vi "form_send_command.vi"(11 "JSON":string) -> ()   [LabVIEW 2021]
doc: "Form for sinding a command."
uses:
  core/host_global_vars.vi
panel:
  in  "command":string
  in  "send button":bool
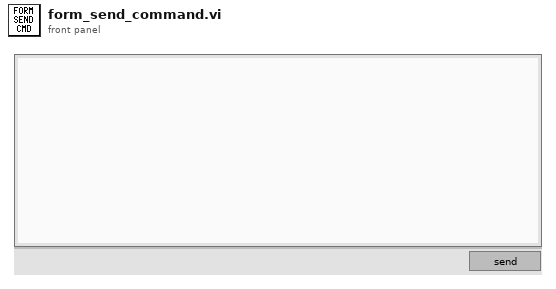
[diagram p1: front panel]
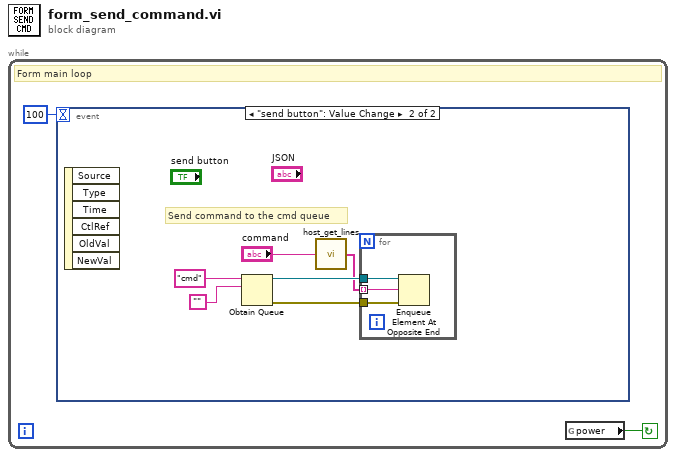
[diagram p0: block diagram]
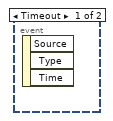
[diagram p2: hidden frame]
diagram:
  n1 = while {
    stop <- w2 continue-if-true
    # "Form main loop"
    n2 = event shown="[1] \"send button\": Value Change" {
      selector: _ -> [_ _]
      dyn-events: _ -> [_ _]
      timeout: 100 -> [_ _]
      event Timeout {
        n3 = event-data() -> ()  [unwired: 1 in, 3 out]
      }
      event "send button": Value Change {
        # "Send command to the cmd queue"
        n4 = event-data() -> ()  [unwired: 1 in, 6 out]
        n5 = Obtain Queue(name (unnamed)="cmd", element data type="") -> (queue out=w6:refnum<queue>, error out=w5:errorcluster)  [unwired: 3 in, 1 out]
        n6 = call "host_get_lines.vi"("in"="command") -> ("out"=w3:string[])
        n7 = for {
          tunnel: w6 -> [w11]
          tunnel: w5 -> [w10]
          tunnel: w3 -> [w9] mode=indexing
          n8 = Enqueue Element At Opposite End(queue=w11, element=w9, error in (no error)=w10) -> ()  [unwired: 1 in, 3 out]
        }
      }
    }
    n9 = global read "host_global_vars.vi" "power"() -> (w2:bool)
  }
